vi "Read MXN.vi"(8 "error in (no error)":errorcluster, 11 "LHL Actor in":refnum<class "LHL Actor.lvclass">) -> (0 "error out":errorcluster, 2 "MXN":bool, 3 "LHL Actor out":refnum<class "LHL Actor.lvclass">)   [LabVIEW 2020, in "LHL Actor.lvlib" / "LHL Actor.lvclass"]
uses:
  LHL Actor.lvclass
  LHL Actor.lvclass/LHL Actor.ctl
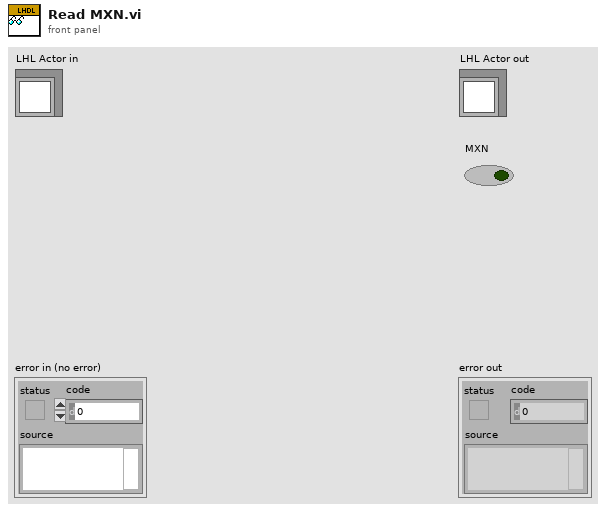
[diagram p1: front panel]
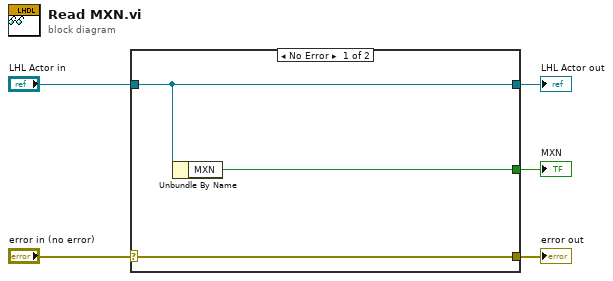
[diagram p0: block diagram]
diagram:
  n1 = case shown="No Error" "error in (no error)" {
    selector: "error in (no error)" -> [w8 w9]
    tunnel: [w8 w9] -> w4
    tunnel: [w7 w10] -> w2
    tunnel: "LHL Actor in" -> [w7 w10]
    tunnel: [w6 _] -> w1
    frame No Error {
      n2 = Unbundle By Name(w7) -> ("MXN"=w6:bool)
    }
    frame Error {
    }
  }
  "error out" <- w4
  "LHL Actor out" <- w2
  "MXN" <- w1
